vi "Check Stream Status.vi"(0 "Register Bus":T1, 1 "scope":string(combo)="rx", 11 "error in":errorcluster) -> (4 "Register Bus (out)":T1, 15 "error out":errorcluster)   [LabVIEW 2017]
doc: "Query the device's stream status. Query the device's stream and data for overflows/underflows, then query for any CLIP/adapter module errors. The stream status should be queried after each Fetch Rx Data/Write Tx Data.\n\n<B>Input Parameters</B>\n\n<B>Register Bus</B> The Register Bus object created by the ni579x Open VI and used as the session handle for the NI-579x Configuration Design Library.\n\n<B>scope</B> is the channel to check the stream status for. The options are \"rx\" and \"tx\".\n\n<B>error in</B> describes error conditions that occur before this node runs. This input provides standard 'error in' functionality.\n\n<B>Output Parameters</B>\n\n<B>Register Bus (out)</B> The Register Bus object created by the ni579x Open VI and used as the session handle for the NI-579x Configuration Design Library.\n\n<B>error out</B> contains error information. This output provides standard 'error out' functionality."
uses:
  <instrlib>/_niInstr/Register Bus/v0/Host/Public/Register Bus Session.ctl
  <instrlib>/_niInstr/Register Bus/v0/Host/Private/Session Data.ctl
  Tx FPGA VI Reference.ctl
  Rx FPGA VI Reference.ctl
  <vilib>/rvi/errors/niLvFpgaAdjustHostInterfaceError.vi
  <vilib>/rvi/interface/nirviReadWriteControl/nirviReadWriteControl.xnode
  <instrlib>/ni579x/Config/v2/Host/ni579x Config v2 Host.lvlib
  NiFpgaLv.dll
  <vilib>/rvi/interface/Simulation/niFpgaSimulationCallBeginRW.vi
  <instrlib>/_niInstr/Register Bus/v0/Host/niInstr Register Bus v0 Host.lvlib
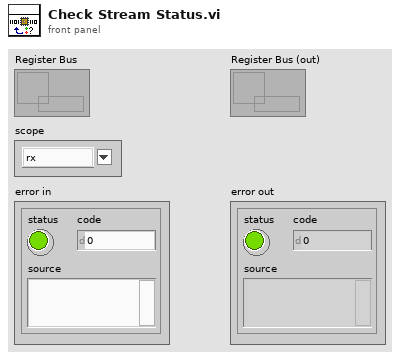
[diagram p1: front panel]
types:
  T1 = typedef "niInstr Register Bus v0 Host.lvlib/Register Bus Session.ctl" = refnum<queue>
  T2 = typedef "Tx FPGA VI Reference.ctl" = refnum<k20>
  T3 = typedef "Rx FPGA VI Reference.ctl" = refnum<k20>
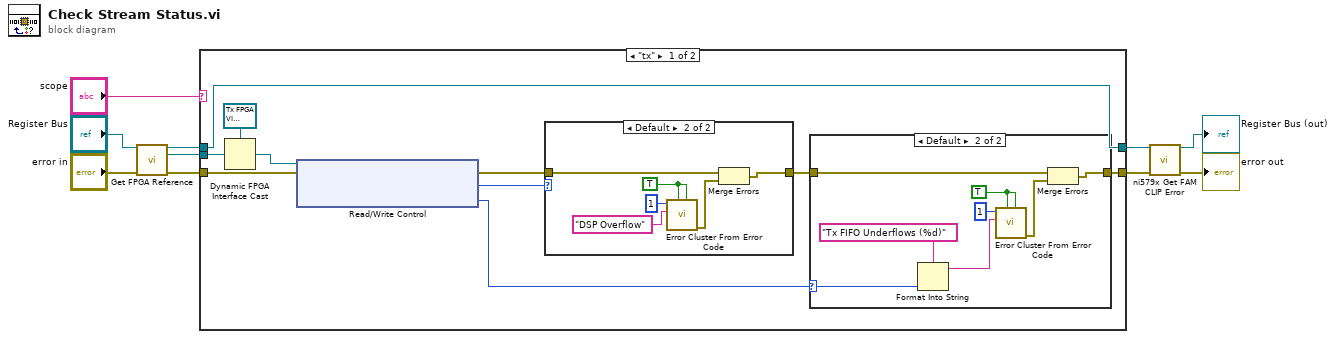
[diagram p0: block diagram]
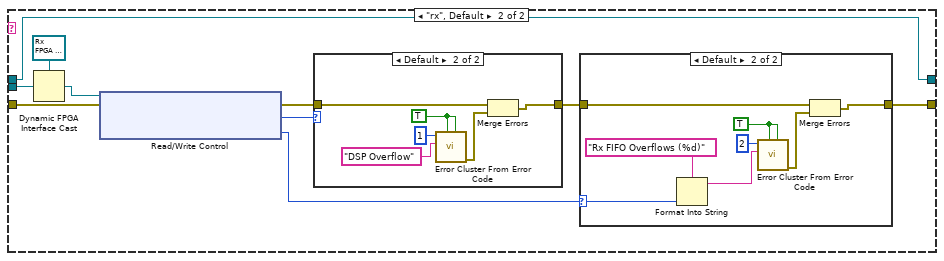
[diagram p4: hidden frame]
diagram:
  n1 = call <instrlib>:"Get FPGA Reference.vi"("session in"="Register Bus", "error in"="error in") -> ("session out"=w2:T1, "fpga ref"=w9:refnum<k20>, "error out"=w8:errorcluster)  [unwired: 11 in]
  n2 = case shown="\"tx\"" "scope" {
    tunnel: w9 -> [w16 w46]
    tunnel: w8 -> [w17 w44]
    tunnel: [w15 w38] -> w7
    tunnel: w2 -> [w14 w37]
    tunnel: [w14 w37] -> w1
    frame "tx" {
      n3 = Dynamic FPGA Interface Cast(Session In=T2 refnum ("Type"), Type=w16) -> (Session Out=w19:T2)
      n4 = xnode "Read/Write Control"("FPGA VI Reference In"=w19, "error in"=w17) -> ("error out"=w12:errorcluster, "tx.number of IQ data overflows"=w11:u64, "tx.underflows"=w20:u32)  [unwired: 1 out]
      n5 = case shown="Default" w11 {
        tunnel: w12 -> [w21 w25]
        tunnel: [w21 w23] -> w13
        frame 0 {
        }
        frame Default {
          w22 = TRUE ("show call chain? (False)")
          n6 = call <vilib>:"Error Cluster From Error Code.vi"("is warning? (False)"=w22, "show call chain? (False)"=w22, "error message (\"\")"="DSP Overflow" ("error message (\"\")"), "error code (0)"=1) -> ("error out"=w24:errorcluster)  [unwired: 5 in]
          n7 = Merge Errors(w25, w24) -> (w23:errorcluster)
        }
      }
      n8 = case shown="Default" w20 {
        selector: w20 -> [_ w29]
        tunnel: w13 -> [w28 w35]
        tunnel: [w28 w33] -> w15
        frame 0 {
        }
        frame Default {
          w30 = TRUE ("show call chain? (False)")
          n9 = Format Into String(format string="Tx FIFO Underflows (%d)" ("error message (\"\")"), w29) -> (resulting string=w31:string)  [unwired: 2 in, 1 out]
          n10 = call <vilib>:"Error Cluster From Error Code.vi"("is warning? (False)"=w30, "show call chain? (False)"=w30, "error message (\"\")"=w31, "error code (0)"=1) -> ("error out"=w34:errorcluster)  [unwired: 5 in]
          n11 = Merge Errors(w35, w34) -> (w33:errorcluster)
        }
      }
    }
    frame "rx", Default {
      n12 = Dynamic FPGA Interface Cast(Session In=T3 refnum ("Type"), Type=w46) -> (Session Out=w43:T3)
      n13 = xnode "Read/Write Control"("FPGA VI Reference In"=w43, "error in"=w44) -> ("error out"=w45:errorcluster, "rx.number of IQ data overflows"=w40:u64, "rx.number of overflows"=w39:u32)  [unwired: 1 out]
      n14 = case shown="Default" w40 {
        tunnel: w45 -> [w56 w60]
        tunnel: [w56 w58] -> w42
        frame 0 {
        }
        frame Default {
          w57 = TRUE ("show call chain? (False)")
          n15 = call <vilib>:"Error Cluster From Error Code.vi"("is warning? (False)"=w57, "show call chain? (False)"=w57, "error message (\"\")"="DSP Overflow" ("error message (\"\")"), "error code (0)"=1) -> ("error out"=w59:errorcluster)  [unwired: 5 in]
          n16 = Merge Errors(w60, w59) -> (w58:errorcluster)
        }
      }
      n17 = case shown="Default" w39 {
        selector: w39 -> [_ w48]
        tunnel: w42 -> [w47 w54]
        tunnel: [w47 w52] -> w38
        frame 0 {
        }
        frame Default {
          w51 = TRUE ("show call chain? (False)")
          n18 = Format Into String(format string="Rx FIFO Overflows (%d)" ("error message (\"\")"), w48) -> (resulting string=w49:string)  [unwired: 2 in, 1 out]
          n19 = call <vilib>:"Error Cluster From Error Code.vi"("is warning? (False)"=w51, "show call chain? (False)"=w51, "error message (\"\")"=w49, "error code (0)"=2) -> ("error out"=w53:errorcluster)  [unwired: 5 in]
          n20 = Merge Errors(w54, w53) -> (w52:errorcluster)
        }
      }
    }
  }
  n21 = call <instrlib>:"ni579x Get FAM CLIP Error.vi"("Register Bus"=w1, "Error In"=w7) -> ("Register Bus (out)"=→"Register Bus (out)":T1, "Error Out"=→"error out":errorcluster)  [unwired: 12 in]
